vi "Init.vi"(8 "error in":errorcluster, 10 "Array":refnum<class "_ISerializable.lvclass">[](array[class])) -> (0 "error out":errorcluster, 3 "LV-ORM out":refnum<class "LV-ORM.lvclass">)   [LabVIEW 2018, in "LV-ORM.lvclass"]
uses:
  LV-ORM.lvclass
  _Serializable Base Object/_ISerializable.lvclass
  ORM Scripter/ORM Scripter.lvclass
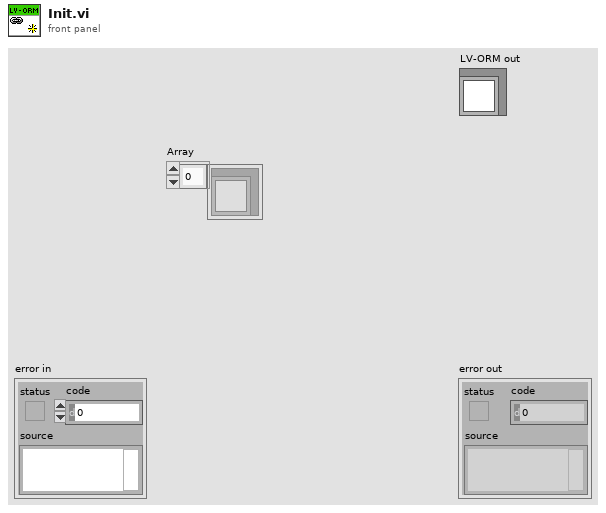
[diagram p1: front panel]
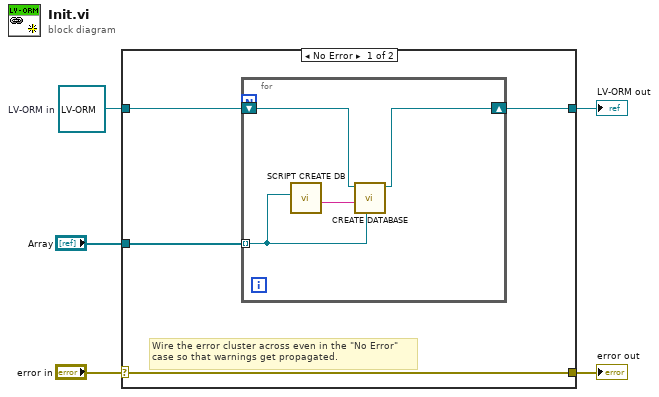
[diagram p0: block diagram]
diagram:
  w3 = refnum<class "LV-ORM.lvclass"> refnum  # LV-ORM in
  n1 = case shown="No Error" "error in" {
    selector: "error in" -> [w9 w15]
    tunnel: [w9 w15] -> w4
    tunnel: [w7 w14] -> w2
    tunnel: w3 -> [w8 w14]
    tunnel: "Array" -> [w6 _]
    frame No Error {
      # "Wire the error cluster across even in the \"No Error\"\ncase so that warnings get propagated."
      n2 = for {
        shift-right: [w11] -> w7
        shift-left: w8 -> [w12]
        tunnel: w6 -> [w10] mode=indexing
        n3 = call "SCRIPT CREATE DB.vi"("class"=w10) -> ("drop-create script"=w13:string)  [unwired: 8 in, 2 out]
        n4 = call "CREATE DATABASE.vi"("object"=w10, "create script 2"=w13, "LV-ORM in"=w12) -> ("LV-ORM out"=w11:refnum<class "LV-ORM.lvclass">)  [unwired: 8 in]
      }
    }
    frame Error {
    }
  }
  "error out" <- w4
  "LV-ORM out" <- w2
